vi "subVI tester.vi"() -> ()   [LabVIEW 2018]
uses:
  <vilib>/Instr/_visa.llb/VISA Configure Serial Port (Instr).vi
panel:
  in  "VISA resource name":refnum<visa-resource-name>="COM9"
  out "sent port 1":string
  out "receive port2":string
  in  "stop":bool
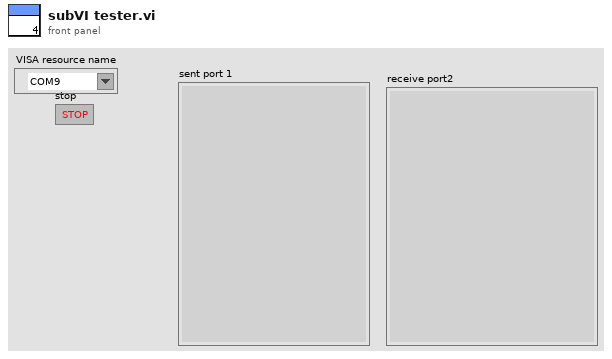
[diagram p1: front panel]
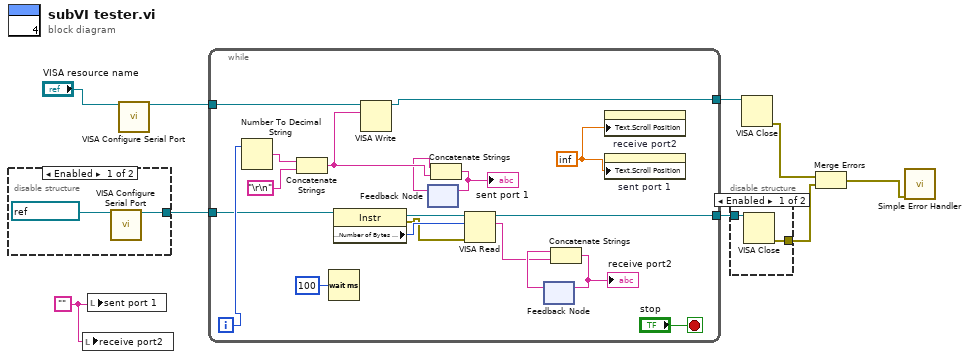
[diagram p0: block diagram]
diagram:
  w1 = ""
  n1 = disable-structure shown="Enabled" {
    disable-tunnel: [w10 _] -> w7
    frame Enabled {
      n2 = call-poly "VISA Configure Serial Port"("VISA resource name"=refnum<visa-resource-name> "COM13") -> ("VISA resource name out"=w10:refnum<visa-resource-name>)  [unwired: 13 in, 1 out]
    }
    frame Disabled {
    }
  }
  n3 = local write "receive port2"(w1) -> ()
  n4 = local write "sent port 1"(w1) -> ()
  n5 = call-poly "VISA Configure Serial Port"("VISA resource name"="VISA resource name") -> ("VISA resource name out"=w8:refnum<visa-resource-name>)  [unwired: 13 in, 1 out]
  n6 = while {
    tunnel: w8 -> [w14]
    tunnel: w7 -> [w13]
    tunnel: [w26] -> w6
    tunnel: [w12] -> w2
    i -> [w30]
    stop <- "stop" stop-if-true
    w15 = inf
    n7 = Number To Decimal String(number=w30) -> (decimal integer string=w29:string)  [unwired: 1 in]
    n8 = Concatenate Strings(w29, "\r\n") -> (w18:string)
    n9 = Wait (ms)(milliseconds to wait=u32 100) -> ()  [unwired: 1 out]
    n10 = property class="Instr"(reference=w13) -> (reference out=w27:refnum<visa-resource-name>, error out=w21:errorcluster, "Serial Settings:Number of Bytes at Serial Port"=w22:u32)  [unwired: 1 in]
    n11 = VISA Write(VISA resource name=w14, write buffer=w18) -> (VISA resource name out=w26:refnum<visa-resource-name>)  [unwired: 1 in, 2 out]
    n12 = feedback #1() -> (w17:string)  [unwired: 1 in]
    n13 = Concatenate Strings(w17, w18) -> (w16:string)
    "sent port 1" <- w16
    n14 = feedback-in #1(w16) -> ()
    n15 = VISA Read(VISA resource name=w27, byte count=w22, error in (no error)=w21) -> (VISA resource name out=w12:refnum<visa-resource-name>, read buffer=w23:string)  [unwired: 2 out]
    n16 = feedback #2() -> (w24:string)  [unwired: 1 in]
    n17 = Concatenate Strings(w24, w23) -> (w25:string)
    "receive port2" <- w25
    n18 = feedback-in #2(w25) -> ()
    n19 = property on="receive port2" class="Str"("Text.Scroll Position"=w15) -> ()  [unwired: 2 in, 2 out]
    n20 = property on="sent port 1" class="Str"("Text.Scroll Position"=w15) -> ()  [unwired: 2 in, 2 out]
  }
  n21 = disable-structure shown="Enabled" {
    disable-tunnel: [w32 _] -> w4
    disable-tunnel: w2 -> [w31 _]
    frame Enabled {
      n22 = VISA Close(VISA resource name=w31) -> (error out=w32:errorcluster)  [unwired: 1 in]
    }
    frame Disabled {
    }
  }
  n23 = VISA Close(VISA resource name=w6) -> (error out=w5:errorcluster)  [unwired: 1 in]
  n24 = Merge Errors(w5, w4) -> (w3:errorcluster)
  n25 = call <vilib>:"Simple Error Handler.vi"("error in (no error)"=w3) -> ()  [unwired: 4 in, 5 out]
